vi "Set Related Enable Pin.vi"(7 "E?E1:E2":bool, 8 "data":bool, 10 "E2":refnum<k21>="E2", 11 "E1":refnum<k21>="E1") -> ()   [LabVIEW 2017, in "HD44780 FPGA.lvlib"]
uses:
  HD44780 FPGA.lvlib
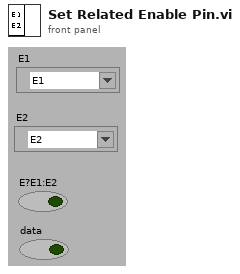
[diagram p1: front panel]
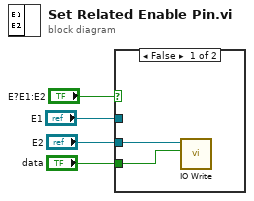
[diagram p0: block diagram]
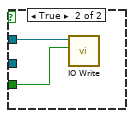
[diagram p2: hidden frame]
diagram:
  n1 = case shown="False" "E?E1:E2" {
    tunnel: "data" -> [w6 w8]
    tunnel: "E2" -> [w5 _]
    tunnel: "E1" -> [_ w7]
    frame False {
      n2 = call "IO Write.vi"("data"=w6, "I/O"=w5) -> ()  [unwired: 10 in]
    }
    frame True {
      n3 = call "IO Write.vi"("data"=w8, "I/O"=w7) -> ()  [unwired: 10 in]
    }
  }
